vi "Core Running.vi"(8 "error in (no error)":errorcluster, 11 "CIFCorePlugin in":refnum<class "CIFCorePlugin.lvclass">) -> (0 "error out":errorcluster, 2 "Destroy":bool, 3 "CIFCorePlugin out":refnum<class "CIFCorePlugin.lvclass">)   [LabVIEW 2021, in "CIFCorePlugin.lvclass"]
doc: "This VI is the main, high priority, execution code. It may be called inside a timed structure. If it is configured to run outside a timed structure, the priority and execution system can be tuned by changing the settings of this VI."
uses:
  CIFCorePlugin.lvclass
  CIFCorePlugin.lvclass/CIFCorePlugin.ctl
  <vilib>/CIF Foundation/CIF Utilities/Statistics/I64/Stats_I64_CIF_U.lvclass/Stats_I64_CIF_U.ctl
  Channels/CIFChannelMng/CIFChannelMng.lvclass/CIFChannelMng.ctl
  Typedef/Energized States.ctl
  <vilib>/CIF Foundation/CIF Utilities/Time/System Time/Sleep Until Future Time.vi
  <vilib>/CIF Foundation/CIF Utilities/Time/System Time/Get System Time.vi
  SubVIs/Timing/Sleep.vi
  Benchmarking/Benchmark Running.vi
  Benchmarking/Benchmark Housekeeping.vi
  SubVIs/OOB/Update Status from Benchmarks.vi
  Channels/CIFChannelMng/Core/Send Channel List Update.vi
  SubVIs/OOB/Send Core OOB TX.vi/074d8088-3ad4-4fdc-9542-b009f1b06b72.vi
  <vilib>/CIF Foundation/CIF Utilities/Time/SubVIs/Add Error.vi
  Accessors/Timestamps/Write Execute TS.vi
  <vilib>/Utility/error.llb/Clear Errors.vi
  Accessors/Read Sleep Limits (ns).vi
  Accessors/Timestamps/Write Target Wake TS.vi
  Accessors/Read Plugin Name.vi
  Common/Utilities/Add Error.vi
  Accessors/Timestamps/Read Running TS.vi
  Accessors/Timestamps/Write Sleep TS.vi
  Benchmarking/Reset Delay.vi
  Accessors/Read Running Internal Data.vi
  Accessors/Read Timing Override.vi
  Accessors/Read Common Config.vi
  Benchmarking/Benchmark Execute.vi
  Accessors/Timestamps/Write Housekeeping TS.vi
  <vilib>/CIF Foundation/CIF Utilities/Statistics/I64/X1 minus X0.vi
  Accessors/Timestamps/Read Housekeeping TS.vi
  <vilib>/CIF Foundation/CIF Utilities/Statistics/I64/Get Stats.vi
  Channels/CIFChannelMng/Core/Send Channel List Update.vi/463ebf4c-8748-40f9-8ad3-9e61c16a01a6.vi
  <vilib>/CIF Foundation/CIF CIPC/SubVIs/Check Error.vi
  <vilib>/CIF Foundation/CIF CIPC/SubVIs/Notify Of New Write.vi
  <vilib>/CIF Foundation/CIF CIPC/SubVIs/Get dll Path.vi
  <vilib>/CIF Foundation/CIF CIPC/SubVIs/Get Element Write Position.vi
  <vilib>/CIF Foundation/CIF Utilities/Errors/Append Error Location.vi
  <vilib>/CIF Foundation/CIF Utilities/Statistics/I64/Cyclic.vi
  Accessors/Timestamps/Read Execute TS.vi
  Accessors/Timestamps/Read Sleep TS.vi
  Accessors/Timestamps/Read Target Wake TS.vi
  <vilib>/CIF Foundation/CIF Utilities/Statistics/I64/X1 minus X0.vi/dfabcf33-0dbc-4041-80a5-3dc0c86d2989.vi
  <vilib>/CIF Foundation/CIF Utilities/Statistics/I64/Cyclic.vi/dfabcf33-0dbc-4041-80a5-3dc0c86d2989.vi
  <vilib>/CIF Foundation/CIF Utilities/Statistics/I64/X1 minus X0.vi/dfabcf33-0dbc-4041-80a5-3dc0c86d2989.vi/9eb60a9a-770f-4d2d-8b3f-8465c267ecc9.vi
  <vilib>/CIF Foundation/CIF Utilities/Statistics/I64/Cyclic.vi/dfabcf33-0dbc-4041-80a5-3dc0c86d2989.vi/9eb60a9a-770f-4d2d-8b3f-8465c267ecc9.vi
  <vilib>/CIF Foundation/CIF CIPC/SubVIs/Get Element Info Variant.vi
  <vilib>/Utility/error.llb/Trim Whitespace.vi
  <vilib>/Utility/error.llb/Error Cluster From Error Code.vi
  SubVIs/OOB/Read Core OOB RX.vi
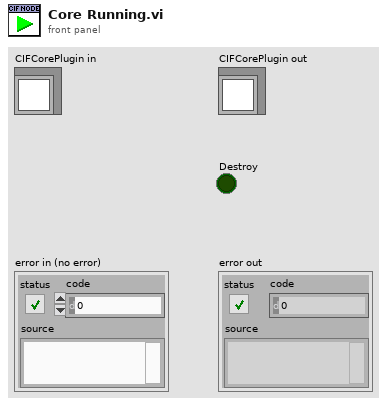
[diagram p1: front panel]
types:
  T1 = typedef "CIFCorePlugin.lvclass/Energized States.ctl" = enum16{"Listen", "Prepare", "Execute", "Housekeep", "Cleanup", "Destroy"}
  T2 = typedef "CIFCorePlugin.lvclass/Running State Logic.ctl" = enum16{"Execute", "Housekeep", "Cleanup", "Error", "Destroy"}
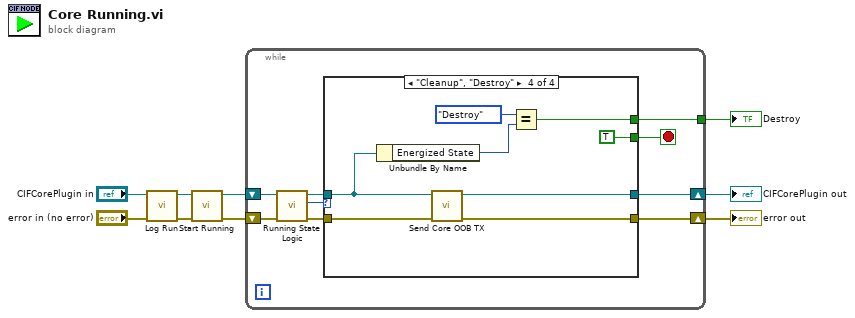
[diagram p0: block diagram]
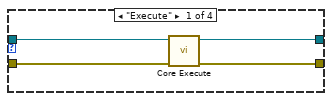
[diagram p2: hidden frame]
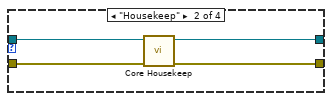
[diagram p3: hidden frame]
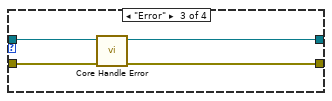
[diagram p4: hidden frame]
diagram:
  n1 = call "Log Run.vi"("error in (no error)"="error in (no error)", "CIFCorePlugin in"="CIFCorePlugin in") -> ("error out"=w2:errorcluster, "CIFCorePlugin out"=w1:refnum<class "CIFCorePlugin.lvclass">)  [unwired: 8 in]
  n2 = call "Start Running.vi"("error in (no error)"=w2, "CIFCorePlugin in"=w1) -> ("error out"=w5:errorcluster, "CIFCorePlugin out"=w6:refnum<class "CIFCorePlugin.lvclass">)  [unwired: 8 in]
  n3 = while {
    shift-right: [w13] -> w8
    shift-left: w6 -> [w18]
    shift-right: [w12] -> w7
    shift-left: w5 -> [w17]
    tunnel: [w10] -> w9
    stop <- w11 stop-if-true
    n4 = call "Running State Logic.vi"("error in (no error)"=w17, "CIFCorePlugin in"=w18) -> ("error out"=w14:errorcluster, "Running State Logic"=w16:T2, "CIFCorePlugin out"=w15:refnum<class "CIFCorePlugin.lvclass">)  [unwired: 7 in]
    n5 = case shown="\"Cleanup\", \"Destroy\"" w16 {
      tunnel: w15 -> [w19 w26 w30 w34]
      tunnel: w14 -> [w22 w25 w29 w37]
      tunnel: [w20 w24 w28 w36] -> w13
      tunnel: [w21 w23 w27 w35] -> w12
      tunnel: [_ _ _ TRUE] -> w11
      tunnel: [_ _ _ w31] -> w10
      frame "Execute" {
        n6 = call "Core Execute.vi"("error in (no error)"=w22, "CIFTemplateNode in"=w19) -> ("error out"=w21:errorcluster, "CIFTemplateNode out"=w20:refnum<class "CIFCorePlugin.lvclass">)  [unwired: 8 in]
      }
      frame "Housekeep" {
        n7 = call "Core Housekeep.vi"("error in (no error)"=w25, "CIFCorePlugin in"=w26) -> ("error out"=w23:errorcluster, "CIFCorePlugin out"=w24:refnum<class "CIFCorePlugin.lvclass">)  [unwired: 8 in]
      }
      frame "Error" {
        n8 = call "Core Handle Error.vi"("error in (no error)"=w29, "CIFTemplateNode in"=w30) -> ("error out"=w27:errorcluster, "CIFTemplateNode out"=w28:refnum<class "CIFCorePlugin.lvclass">)  [unwired: 8 in]
      }
      frame "Cleanup", "Destroy" {
        n9 = Unbundle By Name(w34) -> ("Energized State"=w33:T1)
        n10 = call "Send Core OOB TX.vi"("error in (no error)"=w37, "CIFCorePlugin in"=w34) -> ("error out"=w35:errorcluster, "CIFCorePlugin out"=w36:refnum<class "CIFCorePlugin.lvclass">)  [unwired: 8 in]
        n11 = Equal?(x=Energized_States."Destroy", y=w33) -> (x = y?=w31:bool)
      }
    }
  }
  "error out" <- w7
  "CIFCorePlugin out" <- w8
  "Destroy" <- w9
